vi "Create Tx.vi"(8 "error in (no error)":errorcluster, 11 "RxTx in":refnum<class "CM_RxTx.lvclass">) -> (0 "error out":errorcluster, 3 "RxTx out":refnum<class "CM_RxTx.lvclass">)   [LabVIEW 2018, in "CM_RxTx.lvclass"]
doc: "Create Tx qeue"
uses:
  CM_RxTx.lvclass
  CM_RxTx.lvclass/CM_RxTx.ctl
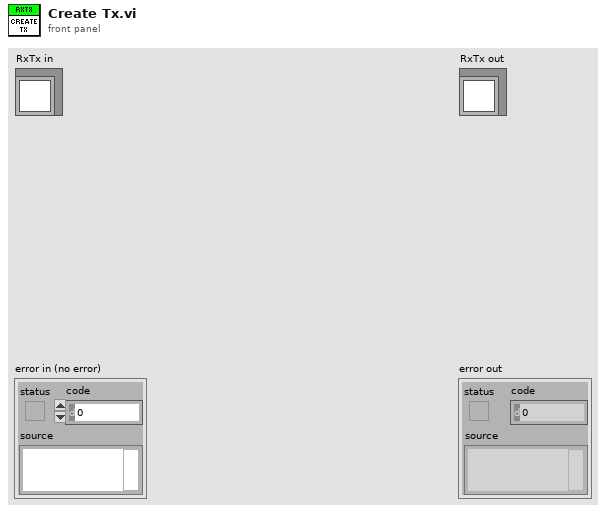
[diagram p1: front panel]
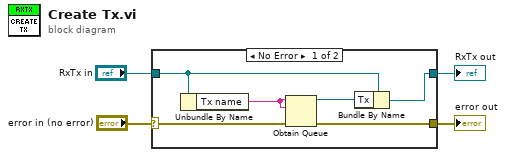
[diagram p0: block diagram]
diagram:
  n1 = case shown="No Error" "error in (no error)" {
    selector: "error in (no error)" -> [w9 w12]
    tunnel: [w10 w12] -> w2
    tunnel: [w8 w11] -> w1
    tunnel: "RxTx in" -> [w6 w11]
    frame No Error {
      n2 = Unbundle By Name(w6) -> ("Tx name"=w5:string)
      n3 = Obtain Queue(name (unnamed)=w5, element data type=w5, error in (no error)=w9) -> (queue out=w7:refnum<queue>, error out=w10:errorcluster)  [unwired: 2 in, 1 out]
      n4 = Bundle By Name(cluster=w6, "Tx"=w7) -> (w8:refnum<class "CM_RxTx.lvclass">)
    }
    frame Error {
    }
  }
  "error out" <- w2
  "RxTx out" <- w1
